vi "Begin.vi"(8 "error in (no error)":errorcluster, 10 "Configuration In":variant, 11 "Cargo Concrete in":refnum<class "Cargo Concrete.lvclass">) -> (0 "error out":errorcluster, 3 "Cargo Concrete out":refnum<class "Cargo Concrete.lvclass">)   [LabVIEW 2019, in "Cargo.lvlib" / "Cargo Concrete.lvclass"]
doc: "Opens resources for cargo motors."
uses:
  Cargo Concrete.lvclass
  Cargo Concrete.lvclass/Cargo Concrete.ctl
  1db68cbf-c77a-4ba6-9063-a73d4232c498.vi
  5e0de1c6-1b8b-49ba-a1ac-9c5146be3bb1.vi
  <vilib>/Utility/error.llb/Trim Whitespace.vi
  <vilib>/Utility/error.llb/Error Cluster From Error Code.vi
  <vilib>/Rock Robotics/WPI/MotorControl/WPI_MotorControlOpen VictorSP.vi
  Cargo.lvclass
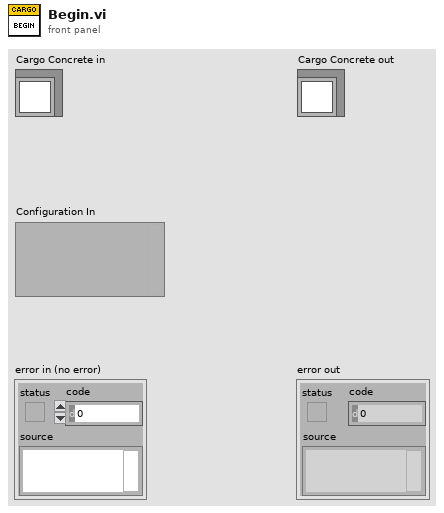
[diagram p1: front panel]
types:
  T1 = typedef "WPI_MotorControlDeviceRef.ctl" = cluster{"DeviceStatus":errorcluster, "Type":T2, "PWM":cluster{"PWM Channel":T3, "DeadBand":T4}, "CAN":cluster{"Device Number":u8, "SetOutput VI Ref":variant, "GetOutput VI Ref":variant, "Enable VI Ref":variant, "Disable VI Ref":variant, "Data":variant}, "Invert":bool, "DIO PWM":cluster{"PWM \"Enable\" Channel":T3, "DIOChannel":T5, "PWM Rate":dbl}}
  T2 = typedef "WPI_MotorControlType.ctl" = enum16{"PWM", "CAN", "DIO PWM"}
  T3 = typedef "FPGA_DIOPWMChannel.ctl" = enum8{"PWM 0", "PWM 1", "PWM 2", "PWM 3", "PWM 4", "PWM 5", "PWM 6", "PWM 7", "PWM 8", "PWM 9", "PWM MXP 0", "PWM MXP 1", "PWM MXP 2", "PWM MXP 3", "PWM MXP 4", "PWM MXP 5", "PWM MXP 6", "PWM MXP 7", "PWM MXP 8", "PWM MXP 9", "Invalid"}
  T4 = typedef "WPI_PWMDeadband.ctl" = cluster{"Name":string, "maxPositivePwm":i32, "minPositivePwm":i32, "centerPwm":i32, "maxNegativePwm":i32, "minNegativePwm":i32, "angularRange":u16}
  T5 = typedef "FPGA_DIOChannel.ctl" = enum8{"DIO 0", "DIO 1", "DIO 2", "DIO 3", "DIO 4", "DIO 5", "DIO 6", "DIO 7", "DIO 8", "DIO 9", "DIO MXP 0", "DIO MXP 1", "DIO MXP 2", "DIO MXP 3", "DIO MXP 4", "DIO MXP 5", "DIO MXP 6", "DIO MXP 7", "DIO MXP 8", "DIO MXP 9", "DIO MXP 10", "DIO MXP 11", "DIO MXP 12", "DIO MXP 13", "DIO MXP 14", "DIO MXP 15", "SPI Port CS1", "SPI Port CS2", "SPI Port CS3", "SPI Port MISO", "SPI Port MOSI", "Invalid"}
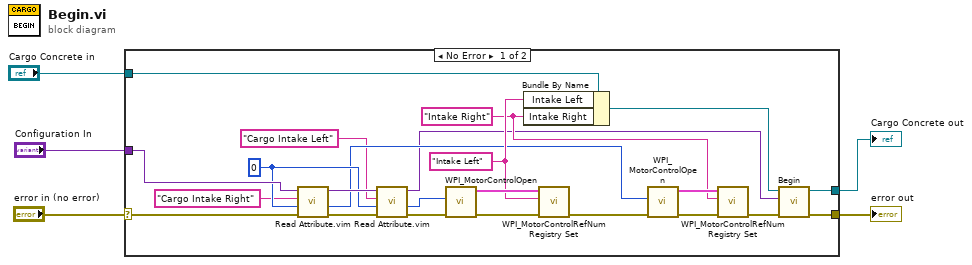
[diagram p0: block diagram]
diagram:
  n1 = case shown="No Error" "error in (no error)" {
    selector: "error in (no error)" -> [w13 w30]
    tunnel: [w28 w30] -> w5
    tunnel: [w27 w29] -> w4
    tunnel: "Cargo Concrete in" -> [w17 w29]
    tunnel: "Configuration In" -> [w14 _]
    frame No Error {
      w11 = u8 0
      w18 = "Intake Right" ("refnum name")
      w19 = "Intake Left" ("refnum name")
      n2 = call "Read Attribute.vim"("error in"=w13, "default value (data type)"=w11, "name"="Cargo Intake Right", "variant in"=w14) -> ("error out"=w16:errorcluster, "value"=w9:u8, "variant out"=w15:variant)  [unwired: 4 in, 1 out]
      n3 = call "Read Attribute.vim"("error in"=w16, "default value (data type)"=w11, "name"="Cargo Intake Left", "variant in"=w15) -> ("error out"=w12:errorcluster, "value"=w10:u8, "variant out"=w8:variant)  [unwired: 4 in, 1 out]
      n4 = call-poly <vilib>:"WPI_MotorControlOpen.vi"("error in (no error)"=w12, "PWM Channel"=w10) -> ("error out"=w23:errorcluster, "MotorControlDeviceRef"=w24:T1)  [unwired: 8 in]
      n5 = Bundle By Name(cluster=w17, "Intake Left"=w19, "Intake Right"=w18) -> (w25:refnum<class "Cargo Concrete.lvclass">)
      n6 = call <vilib>:"WPI_MotorControlRefNum Registry Set.vi"("error in (no error)"=w23, "refnum name"=w19, "MotorControlDevRef"=w24) -> ("error out"=w20:errorcluster)  [unwired: 7 in, 1 out]
      n7 = call-poly <vilib>:"WPI_MotorControlOpen.vi"("error in (no error)"=w20, "PWM Channel"=w9) -> ("error out"=w21:errorcluster, "MotorControlDeviceRef"=w22:T1)  [unwired: 8 in]
      n8 = call <vilib>:"WPI_MotorControlRefNum Registry Set.vi"("error in (no error)"=w21, "refnum name"=w18, "MotorControlDevRef"=w22) -> ("error out"=w26:errorcluster)  [unwired: 7 in, 1 out]
      n9 = call-parent "Begin.vi"("error in (no error)"=w26, "Configuration In"=w8, "Cargo in"=w25) -> ("error out"=w28:errorcluster, "Cargo out"=w27:refnum<class "Cargo Concrete.lvclass">)  [unwired: 7 in]
    }
    frame Error {
    }
  }
  "error out" <- w5
  "Cargo Concrete out" <- w4
